vi "Host_Main.vi"() -> ()   [LabVIEW 2019]
panel:
  in  "stop":bool
  in  "LED ON / OFF":bool
  out "Accelerometer Magnitude":dbl
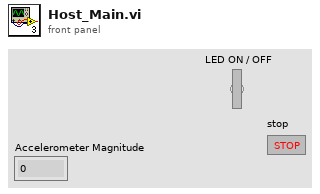
[diagram p1: front panel]
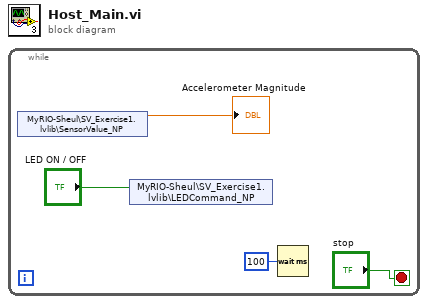
[diagram p0: block diagram]
diagram:
  n1 = while {
    stop <- "stop" stop-if-true
    n2 = shared-variable "MyRIO-Sheul\\SV_Exercise1.lvlib\\SensorValue_NP"() -> (→"Accelerometer Magnitude":dbl)  [unwired: 1 in, 1 out]
    n3 = shared-variable "MyRIO-Sheul\\SV_Exercise1.lvlib\\LEDCommand_NP"("LED ON / OFF") -> ()  [unwired: 1 in, 1 out]
    n4 = Wait (ms)(milliseconds to wait=u32 100) -> ()  [unwired: 1 out]
  }
